vi "RANGE ANSI Calculator.vi"(7 "Meter Number":T1=enum."Meter Bank 3", 8 "Error In":errorcluster, 10 "All Meter Data":T2, 11 "Bank Counter":i32) -> (0 "Error Out":errorcluster, 1 "Count Down Timer":i32, 2 "ANSI Average (BTU/HR)":dbl, 3 "Bank Counter":i32, 5 "Greater than 310 sec":bool)   [LabVIEW 2016]
uses:
  Type Definitions/RANGE DAQ Data Four Meters.ctl
  Type Definitions/RANGE DAQ Data.ctl
  Drivers/Omega FMA-1600A Series Gas Flow Meter/Type Definitions/FMA1600A Gas Type.ctl
  Drivers/Omega FMA-1600A Series Gas Flow Meter/Type Definitions/FMA1600A Units String.ctl
  Type Definitions/RANGE GAS Data.ctl
  Type Definitions/RANGE Panel Data.ctl
  Type Definitions/Range Meter Bank.ctl
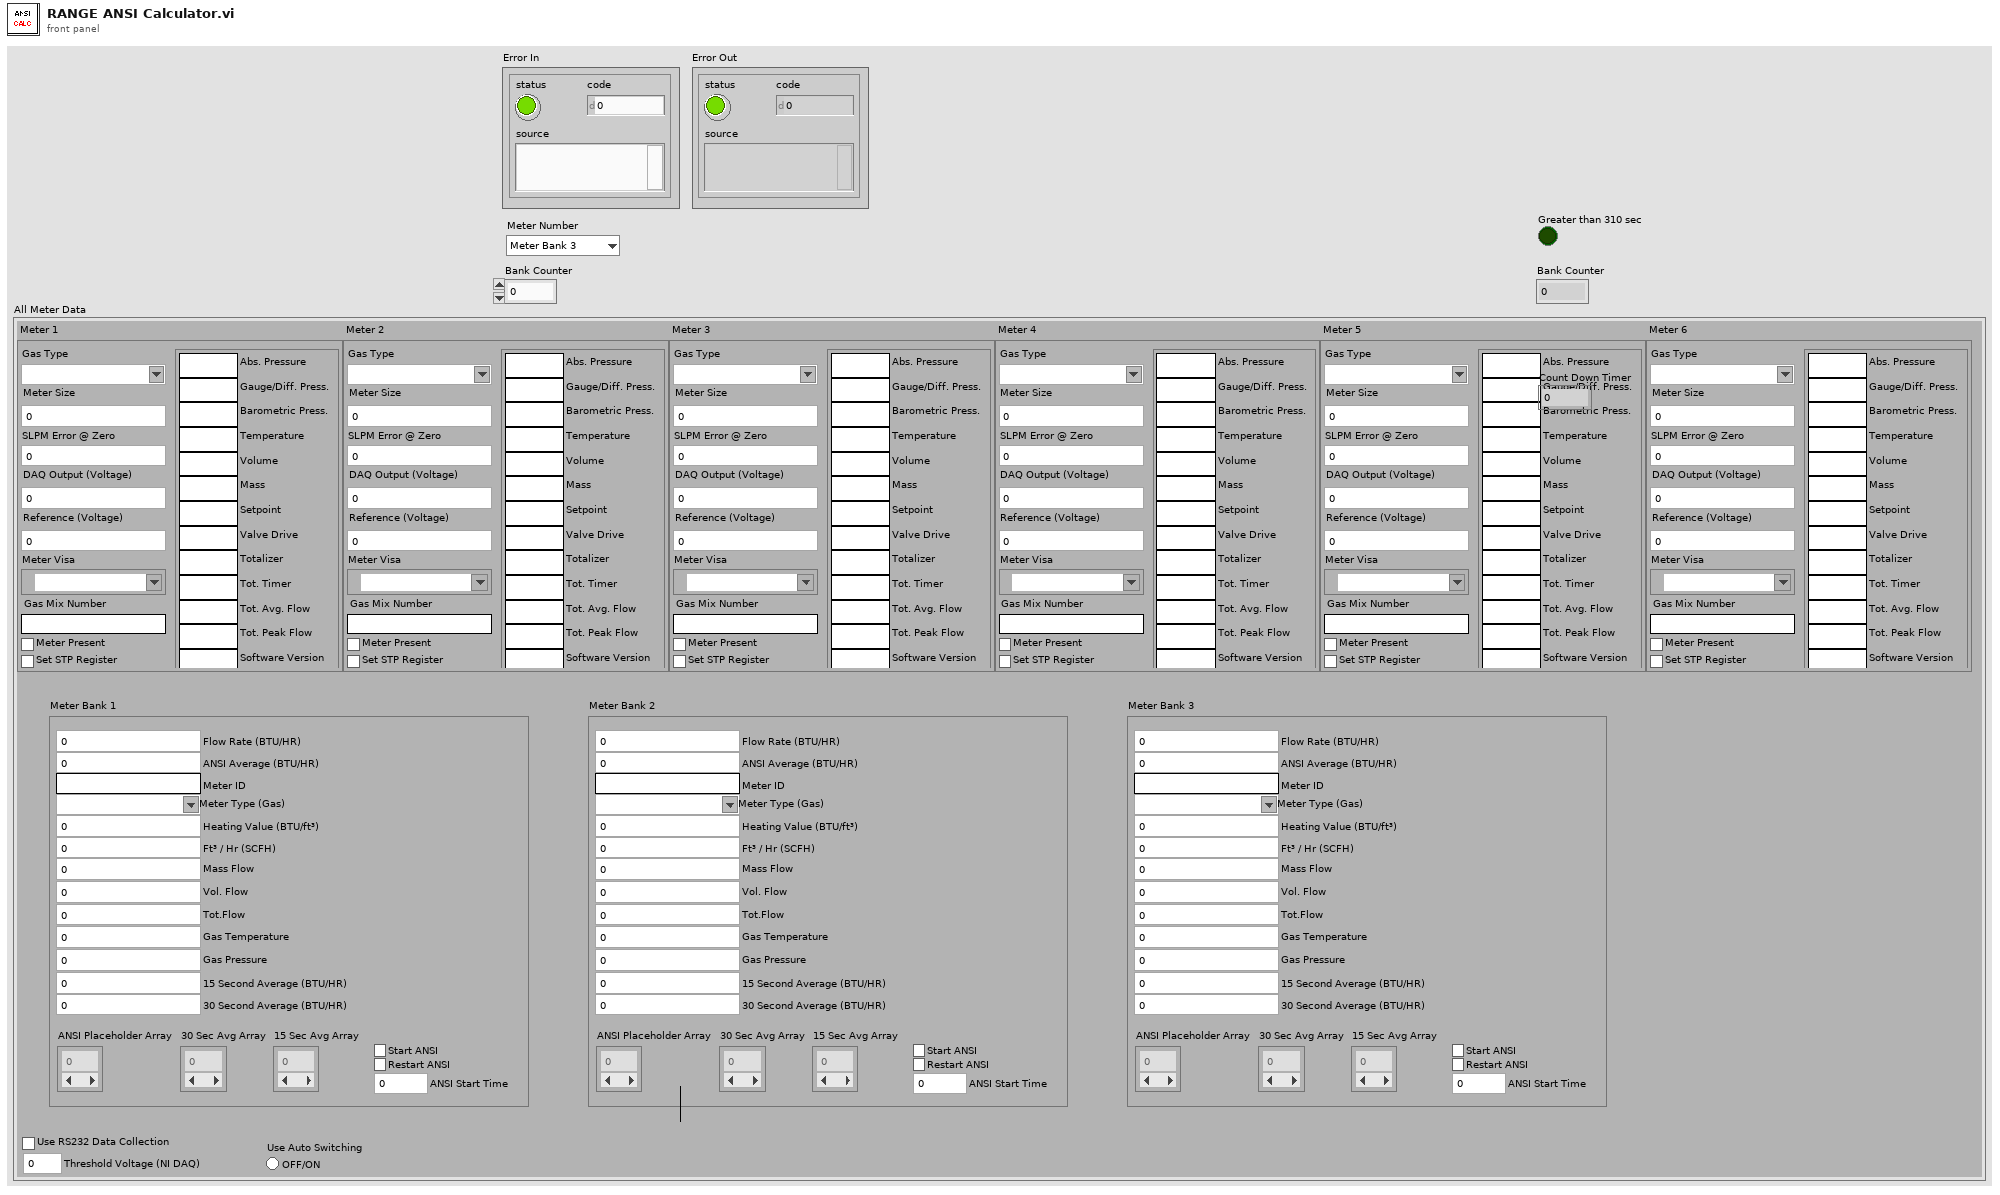
[diagram p1: front panel]
types:
  T1 = typedef "Range Meter Bank.ctl" = enum16{"Meter Bank 1", "Meter Bank 2", "Meter Bank 3"}
  T2 = typedef "RANGE DAQ Data Four Meters.ctl" = cluster{"Meter 1":T3, "Meter 2":T3, "Meter 3":T3, "Meter 4":T3, "Meter 5":T3, "Meter 6":T3, "Meter Bank 1":T6, "Meter Bank 2":T6, "Meter Bank 3":T6, "Threshold Voltage (NI DAQ)":dbl, "Use RS232 Data Collection":bool, "Use Auto Switching":bool}
  T3 = typedef "RANGE DAQ Data.ctl" = cluster{"Meter Size":dbl, "DAQ Output (Voltage)":dbl, "Reference (Voltage)":dbl, "Meter Present":bool, "Meter Visa":refnum<visa-resource-name>, "Gas Type":T4, "SLPM Error @ Zero":dbl, "Gas Mix Number":string, "Set STP Register":bool, "Measurement Units":T5}
  T4 = typedef "FMA1600A Gas Type.ctl" = string
  T5 = typedef "FMA1600A Units String.ctl" = cluster{"Abs. Pressure":string, "Gauge/Diff. Press.":string, "Barometric Press.":string, "Temperature":string, "Volume":string, "Mass":string, "Setpoint":string, "Valve Drive":string, "Totalizer":string, "Tot. Timer":string, "Tot. Avg. Flow":string, "Tot. Peak Flow":string, "Software Version":string}
  T6 = typedef "RANGE GAS Data.ctl" = cluster{"Flow Rate (BTU/HR)":dbl, "ANSI Placeholder Array":dbl[], "15 Sec Avg Array":dbl[], "30 Sec Avg Array ":dbl[], "ANSI Average (BTU/HR)":dbl, "Panel Data":T7, "Start ANSI":bool, "ANSI Start Time":dbl, "Restart ANSI":bool, "Meter ID":string}
  T7 = typedef "RANGE Panel Data.ctl" = cluster{"Meter Type (Gas)":T4, "Heating Value (BTU/ft³)":dbl, "Ft³ / Hr (SCFH)":dbl, "15 Second Average (BTU/HR)":dbl, "30 Second Average (BTU/HR)":dbl, "Mass Flow":dbl, "Vol. Flow":dbl, "Gas Temperature":dbl, "Gas Pressure":dbl, "Tot.Flow":dbl}
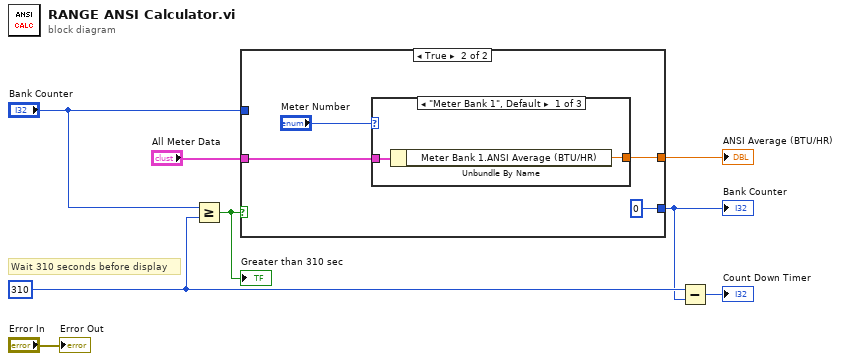
[diagram p0: block diagram]
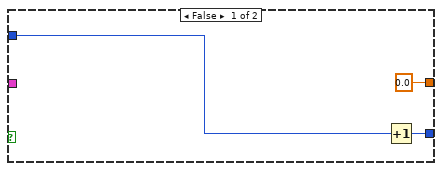
[diagram p2: hidden frame]
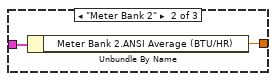
[diagram p3: hidden frame]
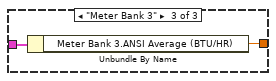
[diagram p4: hidden frame]
diagram:
  w3 = 310 ("y")
  # "Wait 310 seconds before display"
  n1 = Greater Or Equal?(x="Bank Counter", y=w3) -> (x >= y?=w7:bool)
  "Greater than 310 sec" <- w7
  n2 = case shown="True" w7 {
    tunnel: "All Meter Data" -> [_ w15]
    tunnel: [0.0 ("ANSI Average (BTU/HR)") w14] -> w6
    tunnel: "Bank Counter" -> [w11 _]
    tunnel: [w10 0] -> w2
    frame False {
      n3 = Increment(x=w11) -> (x+1=w10:i32)
    }
    frame True {
      n4 = case shown="\"Meter Bank 1\", Default" "Meter Number" {
        tunnel: w15 -> [w17 w19 w21]
        tunnel: [w16 w18 w20] -> w14
        frame "Meter Bank 1", Default {
          n5 = Unbundle By Name(w17) -> ("Meter Bank 1.ANSI Average (BTU/HR)"=w16:dbl)
        }
        frame "Meter Bank 2" {
          n6 = Unbundle By Name(w19) -> ("Meter Bank 2.ANSI Average (BTU/HR)"=w18:dbl)
        }
        frame "Meter Bank 3" {
          n7 = Unbundle By Name(w21) -> ("Meter Bank 3.ANSI Average (BTU/HR)"=w20:dbl)
        }
      }
    }
  }
  "Bank Counter" <- w2
  "ANSI Average (BTU/HR)" <- w6
  n8 = Subtract(x=w3, y=w2) -> (x-y=→"Count Down Timer":i32)
  "Error Out" <- "Error In"
